vi "Configure Trace Operation (Subtract Display Line).vi"(0 "VISA resource name":refnum<visa-resource-name>, 5 "Trace 1 (1: Trace 1)":u16(ring)=1 items=["Trace 1"=1, "Trace 2"=2, "Trace 3"=3], 11 "error in (no error)":errorcluster) -> (4 "VISA resource name out":refnum<visa-resource-name>, 15 "error out":errorcluster)   [LabVIEW 2014, in "Agilent ESA PSA Series.lvlib"]
doc: "Subtracts the magnitude of the display line from the selected trace and places the result back in the selected trace."
uses:
  Agilent ESA PSA Series.lvlib
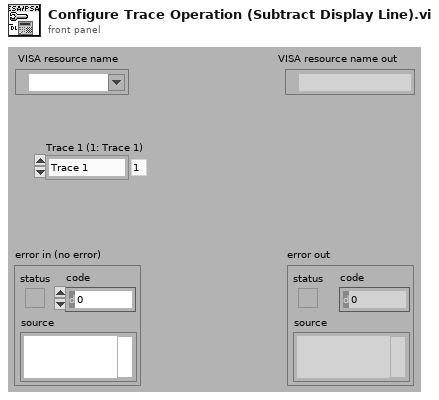
[diagram p1: front panel]
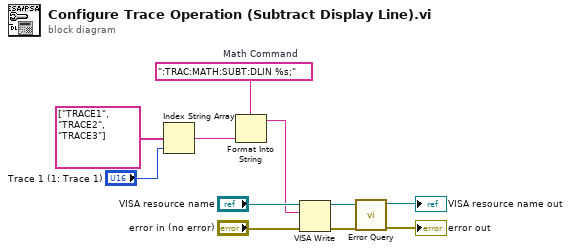
[diagram p0: block diagram]
diagram:
  w3 = ":TRAC:MATH:SUBT:DLIN %s;"  # Math Command
  n1 = Index String Array(1:"Trace 1 (1: Trace 1)", 2:string[] ["TRACE1", "TRACE2", "TRACE3"]) -> (0:w2:string)  [unwired: 1 in]
  n2 = Format Into String(format string=w3, w2) -> (resulting string=w1:string)  [unwired: 2 in, 1 out]
  n3 = VISA Write(VISA resource name="VISA resource name", write buffer=w1, error in (no error)="error in (no error)") -> (VISA resource name out=w9:refnum<visa-resource-name>, error out=w7:errorcluster)  [unwired: 1 out]
  n4 = call "Error Query.vi"("error in (no error)"=w7, "VISA resource name"=w9) -> ("error out"=→"error out":errorcluster, "VISA resource name out"=→"VISA resource name out":refnum<visa-resource-name>)  [unwired: 6 in, 2 out]
